vi "Write Response.vi"(8 "error in (no error)":errorcluster, 10 "Response":string, 11 "T560Channel in":refnum<class "T560Channel.lvclass">) -> (0 "error out":errorcluster, 3 "T560Channel out":refnum<class "T560Channel.lvclass">)   [LabVIEW 2013, in "T560Channel.lvclass"]
uses:
  T560Channel.lvclass
  T560Channel.lvclass/T560Channel.ctl
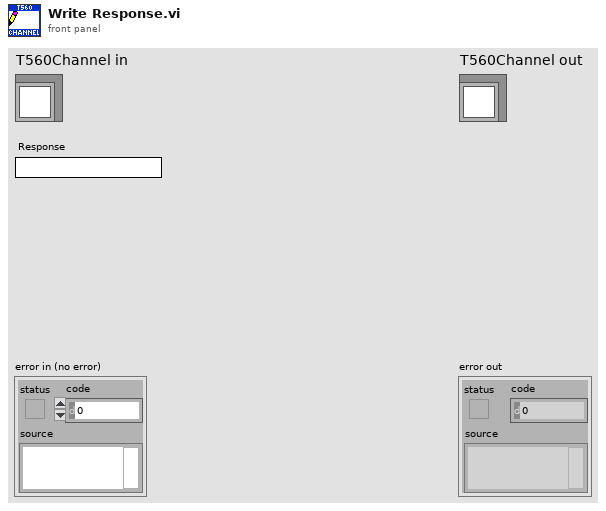
[diagram p1: front panel]
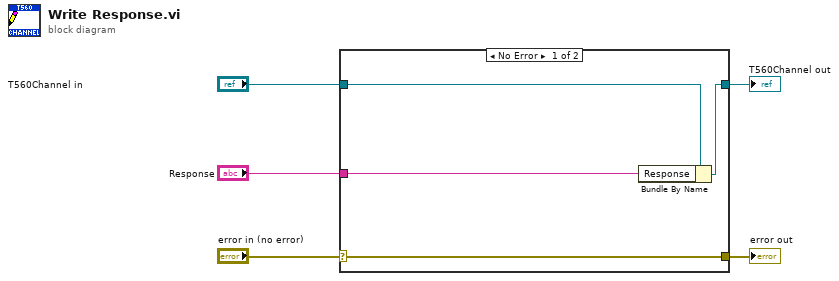
[diagram p0: block diagram]
diagram:
  n1 = case shown="No Error" "error in (no error)" {
    selector: "error in (no error)" -> [w9 w10]
    tunnel: [w9 w10] -> w4
    tunnel: [w7 w11] -> w2
    tunnel: "T560Channel in" -> [w8 w11]
    tunnel: "Response" -> [w6 _]
    frame No Error {
      n2 = Bundle By Name(cluster=w8, "Response"=w6) -> (w7:refnum<class "T560Channel.lvclass">)
    }
    frame Error {
    }
  }
  "error out" <- w4
  "T560Channel out" <- w2
